vi "Serial Port Test.vi"(11 "VISA resource name":refnum<visa-resource-name>="COM1") -> ()   [LabVIEW 2020]
uses:
  <vilib>/Instr/_visa.llb/VISA Configure Serial Port (Instr).vi
panel:
  in  "stop":bool
  out "Receive":string
  out "Response":string
  in  "Send":bool
  in  "Send":string
  in  "VISA resource name 2":refnum<visa-resource-name>="COM1"
  in  "flow control":u16(ring) items=["None"=0, "XON/XOFF"=1, "RTS/CTS"=2, "DTR/DSR"=4]
  in  "stop bits":u16(ring)=10 items=["1.0"=10, "1.5"=15, "2.0"=20]
  in  "parity":u16(ring) items=["None", "Odd", "Even", "Mark", "Space"]
  in  "data bits":u16=8 min=5 max=8 step=1
  in  "baud rate":u32=19200
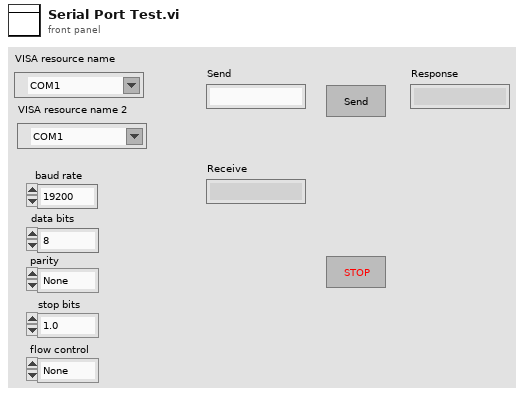
[diagram p1: front panel]
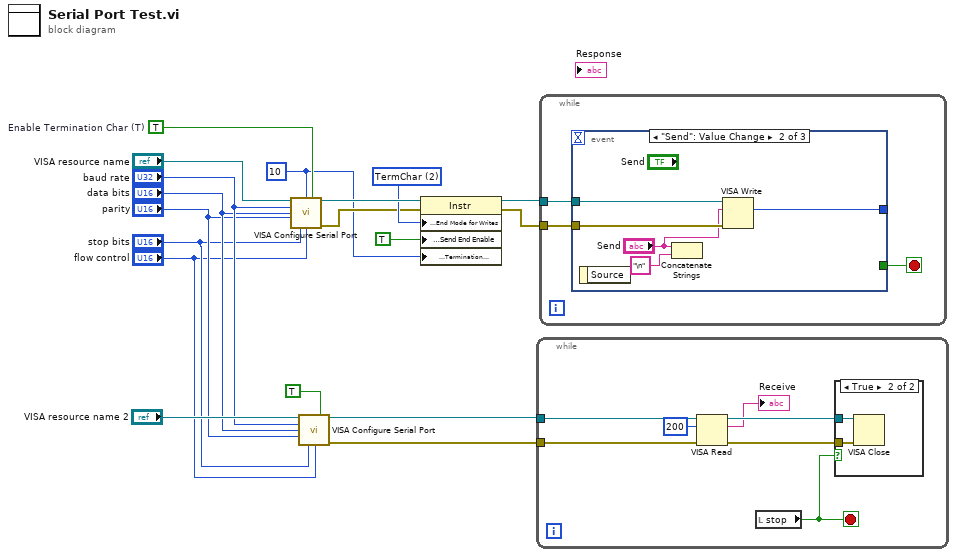
[diagram p0: block diagram]
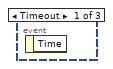
[diagram p3: hidden frame]
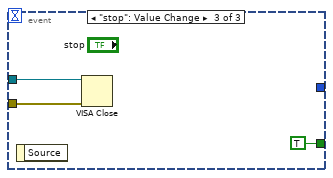
[diagram p4: hidden frame]
diagram:
  w1 = u8 10 ("termination char\n(0xA = '\\n' = LF)")
  w6 = u16 2 items=["None", "LastBit", "TermChar", "Break"] ("Serial Settings:Serial End Mode for Writes")
  w17 = TRUE  # Enable Termination Char (T)
  n1 = call-poly "VISA Configure Serial Port"("VISA resource name"="VISA resource name", "termination char\n(0xA = '\\n' = LF)"=w1, "Enable Termination\nChar (T)"=w17, "baud rate (9600)"="baud rate", "data bits (8)"="data bits", "parity (0:none)"="parity", "stop bits (10: 1 bit)"="stop bits", "flow control (0:none)"="flow control") -> ("VISA resource name out"=w7:refnum<visa-resource-name>, "error out"=w4:errorcluster)  [unwired: 6 in]
  n2 = call-poly "VISA Configure Serial Port"("VISA resource name"="VISA resource name 2", "Enable Termination\nChar (T)"=TRUE ("Enable Termination\nChar (T)"), "baud rate (9600)"="baud rate", "data bits (8)"="data bits", "parity (0:none)"="parity", "stop bits (10: 1 bit)"="stop bits", "flow control (0:none)"="flow control") -> ("VISA resource name out"=w16:refnum<visa-resource-name>, "error out"=w15:errorcluster)  [unwired: 7 in]
  n3 = property class="Instr"(reference=w7, error in=w4, "Serial Settings:End Mode for Writes"=w6, "Message Based Settings:Send End Enable"=TRUE, "Message Based Settings:Termination Character"=w1) -> (reference out=w3:refnum<visa-resource-name>, error out=w2:errorcluster)
  n4 = while {
    tunnel: w16 -> [w21]
    tunnel: w15 -> [w20]
    stop <- w25 stop-if-true
    n5 = VISA Read(VISA resource name=w21, byte count=u32 200, error in (no error)=w20) -> (VISA resource name out=w24:refnum<visa-resource-name>, read buffer=→"Receive":string, error out=w23:errorcluster)  [unwired: 1 out]
    n6 = local read "stop"() -> (w25:bool)
    n7 = case shown="True" w25 {
      tunnel: w24 -> [_ w27]
      tunnel: w23 -> [_ w26]
      frame False {
      }
      frame True {
        n8 = VISA Close(VISA resource name=w27, error in (no error)=w26) -> ()  [unwired: 1 out]
      }
    }
  }
  n9 = while {
    tunnel: w3 -> [w30]
    tunnel: w2 -> [w29]
    stop <- w28 stop-if-true
    n10 = event shown="[1] \"Send\": Value Change" {
      selector: _ -> [_ _ _]
      dyn-events: _ -> [_ _ _]
      timeout: _ -> [_ _ _]
      tunnel: w30 -> [_ w35 w38]
      tunnel: w29 -> [_ w34 w37]
      tunnel: [_ _ TRUE] -> w28
      tunnel: [_ w32 _] -> _
      event Timeout {
        n11 = event-data() -> ()  [unwired: 1 in, 1 out]
      }
      event "Send": Value Change {
        n12 = event-data() -> ()  [unwired: 1 in, 1 out]
        n13 = Concatenate Strings("Send", "\n" ("string")) -> ()  [unwired: 1 out]
        n14 = VISA Write(VISA resource name=w35, write buffer="Send", error in (no error)=w34) -> (return count=w32:u32)  [unwired: 2 out]
      }
      event "stop": Value Change {
        n15 = event-data() -> ()  [unwired: 1 in, 1 out]
        n16 = VISA Close(VISA resource name=w38, error in (no error)=w37) -> ()  [unwired: 1 out]
      }
    }
  }
